vi "Lab15.vi"() -> ()   [LabVIEW 2022 SP3]
uses:
  <vilib>/DAQmx/read.llb/DAQmx Read (Counter 1D DBL 1Chan NSamp).vi
  <vilib>/DAQmx/create/channels.llb/DAQmx Create Channel (CI-Frequency).vi
  <vilib>/DAQmx/configure/timing.llb/DAQmx Timing (Implicit).vi
  <vilib>/DAQmx/miscellaneous.llb/DAQmx Fill In Error Info.vi
  <resource>/objmgr/daqmx.rc
panel:
  out "Measured Frequency":dbl format="%#_6p"
  in  "Samples per \nMeasurement":i32=-1
  in  "CI.Freq.Term":tag
  in  "Counter":tag
  in  "stop":bool
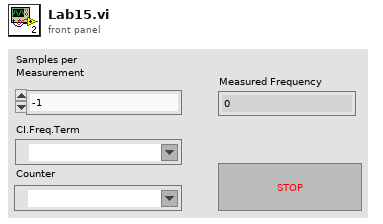
[diagram p1: front panel]
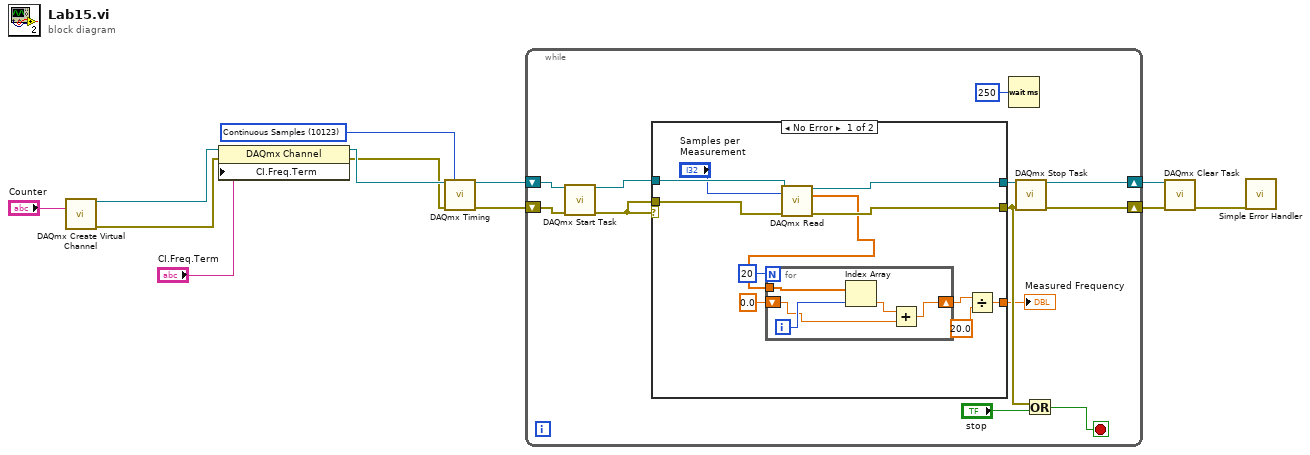
[diagram p0: block diagram]
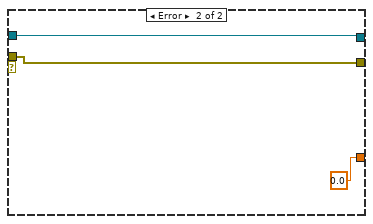
[diagram p2: hidden frame]
diagram:
  w1 = 10123 items=["Finite Samples"=10178, "Continuous Samples"=10123, "Hardware Timed Single Point"=12522] ("sample mode")
  n1 = call-poly <vilib>:"DAQmx Create Virtual Channel.vi"("counter"="Counter") -> ("task out"=w9:refnum<k21>, "error out"=w8:errorcluster)  [unwired: 13 in]
  n2 = property class="DAQmx Channel"(reference=w9, error in=w8, "CI.Freq.Term"="CI.Freq.Term") -> (reference out=w5:refnum<k21>, error out=w4:errorcluster)
  n3 = call-poly <vilib>:"DAQmx Timing.vi"("task/channels in"=w5, "sample mode"=w1, "error in"=w4) -> ("task out"=w3:refnum<k21>, "error out"=w2:errorcluster)  [unwired: 11 in]
  n4 = while {
    shift-right: [w19] -> w7
    shift-left: w3 -> [w17]
    shift-right: [w18] -> w6
    shift-left: w2 -> [w16]
    stop <- w15 stop-if-true
    n5 = call <vilib>:"DAQmx Start Task.vi"("task/channels in"=w17, "error in"=w16) -> ("task out"=w22:refnum<k21>, "error out"=w21:errorcluster)  [unwired: 12 in]
    n6 = case shown="No Error" w21 {
      tunnel: [w35 w43] -> w20
      tunnel: [w34 w42] -> w24
      tunnel: w21 -> [w33 w42]
      tunnel: w22 -> [w32 w43]
      tunnel: [w27 0.0] -> w13
      frame No Error {
        n7 = call-poly <vilib>:"DAQmx Read.vi"("task/channels in"=w32, "number of samples per channel"="Samples per \nMeasurement", "error in"=w33) -> ("task out"=w35:refnum<k21>, "data"=w30:dbl[], "error out"=w34:errorcluster)  [unwired: 10 in]
        n8 = for {
          N: 20 -> [_]
          tunnel: w30 -> [w40]
          shift-right: [w37] -> w25
          shift-left: 0.0 -> [w36]
          i -> [w39]
          n9 = Index Array(array=w40, index=w39) -> (element=w38:dbl)
          n10 = Add(x=w38, y=w36) -> (x+y=w37:dbl)
        }
        n11 = Divide(x=w25, y=20.0) -> (x/y=w27:dbl)
      }
      frame Error {
      }
    }
    "Measured Frequency" <- w13
    n12 = Wait (ms)(milliseconds to wait=u32 250) -> ()  [unwired: 1 out]
    n13 = call <vilib>:"DAQmx Stop Task.vi"("task/channels in"=w20, "error in"=w24) -> ("task out"=w19:refnum<k21>, "error out"=w18:errorcluster)  [unwired: 12 in]
    n14 = Or(x=w24, y="stop") -> (x .or. y?=w15:bool)
  }
  n15 = call <vilib>:"DAQmx Clear Task.vi"("task in"=w7, "error in"=w6) -> ("error out"=w11:errorcluster)  [unwired: 13 in]
  n16 = call <vilib>:"Simple Error Handler.vi"("error in (no error)"=w11) -> ()  [unwired: 4 in, 5 out]
